vi "LENGTH校验计算.vi"(11 "info字节数":u16 format="%xH") -> (3 "LENGTH":u16 format="%xH")   [LabVIEW 2016, in "环境动力监测库.lvlib" / "空调库.lvlib"]
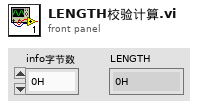
[diagram p1: front panel]
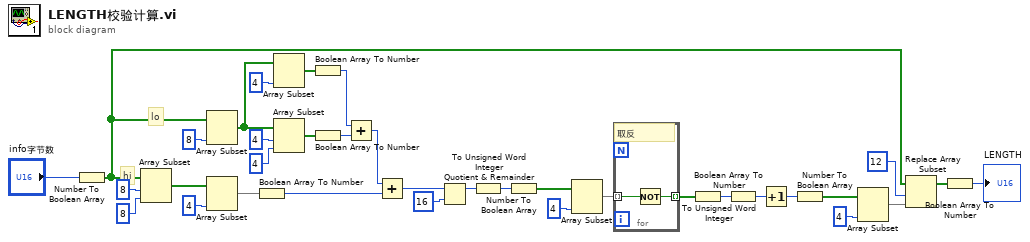
[diagram p0: block diagram]
diagram:
  # "hi"
  # "lo"
  n1 = Number To Boolean Array(number="info字节数") -> (Boolean array=w29:bool[])
  n2 = Array Subset(array=w29, index=8 ("索引"), length=8 ("长度")) -> (w6:bool[])
  n3 = Array Subset(array=w29, length=8 ("长度")) -> (w10:bool[])  [unwired: 1 in]
  n4 = Array Subset(array=w6, length=4 ("长度")) -> (w8:bool[])  [unwired: 1 in]
  n5 = Boolean Array To Number(Boolean array=w8) -> (number=w18:u32)
  n6 = Array Subset(array=w10, length=4 ("长度")) -> (w13:bool[])  [unwired: 1 in]
  n7 = Array Subset(array=w10, index=4 ("索引"), length=4 ("长度")) -> (w14:bool[])
  n8 = Boolean Array To Number(Boolean array=w13) -> (number=w15:u32)
  n9 = Boolean Array To Number(Boolean array=w14) -> (number=w16:u32)
  n10 = Add(x=w15, y=w16) -> (x+y=w17:u32)
  n11 = Add(x=w17, y=w18) -> (x+y=w20:u32)
  n12 = Quotient & Remainder(x=w20, y=u32 16) -> (x-y*floor(x/y)=w21:u32)  [unwired: 1 out]
  n13 = To Unsigned Word Integer(number=w21) -> (unsigned 16bit integer=w22:u16)
  n14 = Number To Boolean Array(number=w22) -> (Boolean array=w27:bool[])
  n15 = Array Subset(array=w27, length=4 ("长度")) -> (w28:bool[])  [unwired: 1 in]
  n16 = for {
    tunnel: w28 -> [w37] mode=indexing
    tunnel: [w36] -> w23 mode=indexing
    # "取反"
    n17 = Not(x=w37) -> (.not. x?=w36:bool)
  }
  n18 = Boolean Array To Number(Boolean array=w23) -> (number=w24:u32)
  n19 = To Unsigned Word Integer(number=w24) -> (unsigned 16bit integer=w25:u16)
  n20 = Increment(x=w25) -> (x+1=w30:u16)
  n21 = Number To Boolean Array(number=w30) -> (Boolean array=w32:bool[])
  n22 = Array Subset(array=w32, length=4 ("长度")) -> (w33:bool[])  [unwired: 1 in]
  n23 = Replace Array Subset(array=w29, new element=w33, index=12 ("索引")) -> (w35:bool[])
  n24 = Boolean Array To Number(Boolean array=w35) -> (number=→"LENGTH":u32)
